vi "Configure channel.vi"(6 "TPC":T2={"Vertical Range (V)"=0.2, "Vertical Offset (0.0 divs)"=0.4, "Bandwidth"=0, "Probe Attenuation (10.0)"=1.0, "Vertical Coupling"=1, "Impedance"=2, "Multiplication factor"=1.0, "Channel"=enum."Channel 1"} {"Impedance" items=["1M", "75", "50"]; "Vertical Coupling" items=["AC", "DC", "Ground"]; "Bandwidth" items=["FULL", "250 MHz", "150 MHz", "20 MHz"]}, 7 "Model":T1=enum."TDS 3012C", 8 "error in (no error)":errorcluster, 11 "VISA Refnum in":refnum<visa-resource-name>) -> (0 "error out":errorcluster, 3 "VISA Refnum out":refnum<visa-resource-name>)   [LabVIEW 2017, in "Scope.lvlib"]
uses:
  Scope.lvlib
  Controls/TPC.ctl
  Controls/Channels.ctl
  Controls/Models.ctl
  Third Party Drivers/Tektronix DPO MSO 2000 4000 Series/Tektronix DPO MSO 2000 4000 Series.lvlib
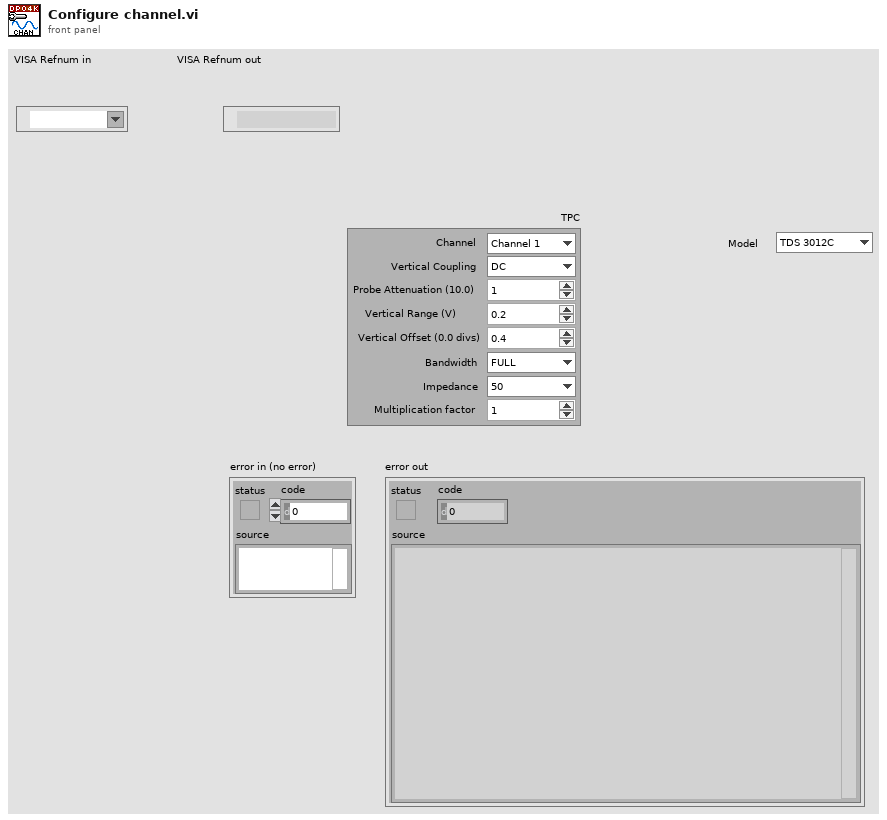
[diagram p1: front panel]
types:
  T1 = typedef "Scope.lvlib/Models.ctl" = enum16{"DPO 3012", "DPO 2012B", "TDS 3012C"}
  T2 = typedef "Scope.lvlib/TPC.ctl" = cluster{"Vertical Range (V)":dbl, "Vertical Offset (0.0 divs)":dbl, "Bandwidth":i32, "Probe Attenuation (10.0)":dbl, "Vertical Coupling":u16, "Impedance":u16, "Multiplication factor":dbl, "Channel":T3}
  T3 = typedef "Scope.lvlib/Channels.ctl" = enum16{"Channel 1", "Channel 2", "Channel 3", "Channel 4", "Math", "Reference A", "Reference B", "Reference C", "Reference D", "B1", "B2", "None"}
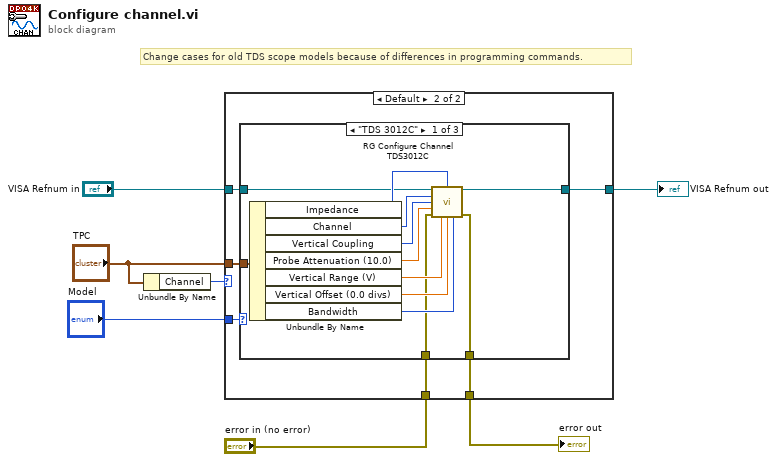
[diagram p0: block diagram]
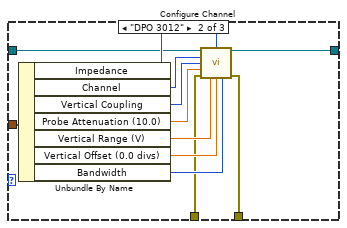
[diagram p3: hidden frame]
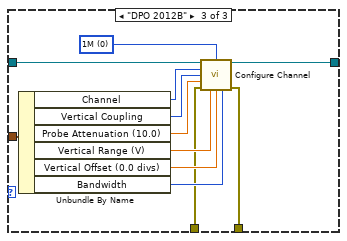
[diagram p4: hidden frame]
diagram:
  # "Change cases for old TDS scope models because of differences in programming commands."
  n1 = Unbundle By Name("TPC") -> ("Channel"=w1:T3)
  n2 = case shown="Default" w1 {
    tunnel: [w9 w15] -> w7
    tunnel: "VISA Refnum in" -> [w9 w14]
    tunnel: "error in (no error)" -> [w8 w13]
    tunnel: [w8 w12] -> w4
    tunnel: "Model" -> [_ w11]
    tunnel: "TPC" -> [_ w10]
    frame "None" {
    }
    frame Default {
      n3 = case shown="\"TDS 3012C\"" w11 {
        tunnel: w10 -> [w20 w32 w45]
        tunnel: [w19 w31 w44] -> w15
        tunnel: w14 -> [w18 w30 w43]
        tunnel: w13 -> [w17 w29 w42]
        tunnel: [w16 w28 w41] -> w12
        frame "TDS 3012C" {
          n4 = Unbundle By Name(w20) -> ("Impedance"=w27:u16, "Channel"=w21:T3, "Vertical Coupling"=w22:u16, "Probe Attenuation (10.0)"=w23:dbl, "Vertical Range (V)"=w24:dbl, "Vertical Offset (0.0 divs)"=w25:dbl, "Bandwidth"=w26:i32)
          n5 = call "RG Configure Channel TDS3012C.vi"("VISA resource name"=w18, "Input Impedance (0: 1M ohm)"=w27, "Channel (0: Channel 1)"=w21, "Vertical Coupling (1: DC)"=w22, "Probe Attenuation (1)"=w23, "error in (no error)"=w17, "Vertical Range (10.0 V)"=w24, "Vertical Offset (0.0 V)"=w25, "Bandwidth (0: FULL)"=w26) -> ("VISA resource name out"=w19:refnum<visa-resource-name>, "error out"=w16:errorcluster)  [unwired: 5 in]
        }
        frame "DPO 3012" {
          n6 = Unbundle By Name(w32) -> ("Impedance"=w39:u16, "Channel"=w33:T3, "Vertical Coupling"=w34:u16, "Probe Attenuation (10.0)"=w35:dbl, "Vertical Range (V)"=w36:dbl, "Vertical Offset (0.0 divs)"=w37:dbl, "Bandwidth"=w38:i32)
          n7 = call "Configure Channel.vi"("VISA resource name"=w30, "Input Impedance (0: 1M ohm)"=w39, "Channel (0: Channel 1)"=w33, "Vertical Coupling (1: DC)"=w34, "Probe Attenuation (1)"=w35, "error in (no error)"=w29, "Vertical Range (10.0 V)"=w36, "Vertical Offset (0.0 V)"=w37, "Bandwidth (0: FULL)"=w38) -> ("VISA resource name out"=w31:refnum<visa-resource-name>, "error out"=w28:errorcluster)  [unwired: 5 in]
        }
        frame "DPO 2012B" {
          w40 = u16 0 items=["1M", "75", "50"] ("Input Impedance (0: 1M ohm)")
          n8 = Unbundle By Name(w45) -> ("Channel"=w46:T3, "Vertical Coupling"=w47:u16, "Probe Attenuation (10.0)"=w48:dbl, "Vertical Range (V)"=w49:dbl, "Vertical Offset (0.0 divs)"=w50:dbl, "Bandwidth"=w51:i32)
          n9 = call "Configure Channel.vi"("VISA resource name"=w43, "Input Impedance (0: 1M ohm)"=w40, "Channel (0: Channel 1)"=w46, "Vertical Coupling (1: DC)"=w47, "Probe Attenuation (1)"=w48, "error in (no error)"=w42, "Vertical Range (10.0 V)"=w49, "Vertical Offset (0.0 V)"=w50, "Bandwidth (0: FULL)"=w51) -> ("VISA resource name out"=w44:refnum<visa-resource-name>, "error out"=w41:errorcluster)  [unwired: 5 in]
        }
      }
    }
  }
  "VISA Refnum out" <- w7
  "error out" <- w4
